vi "process board dll.vi"(8 "error in (no error)":errorcluster, 11 "board":i8) -> (0 "error out":errorcluster, 3 "board out":i8)   [LabVIEW 2025, in "uncoverspace.lvlib"]
doc: "void process_board_dll(int8_t board[Z][Y][X]);\nvoid process_board_dll(int8_t *board);"
uses:
  uncoverspace.lvlib
  uncoverspace.dll
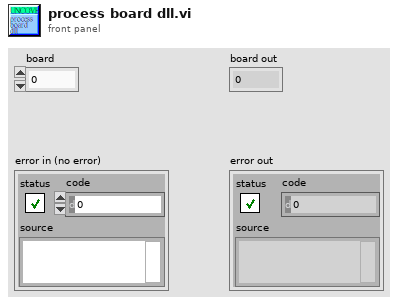
[diagram p1: front panel]
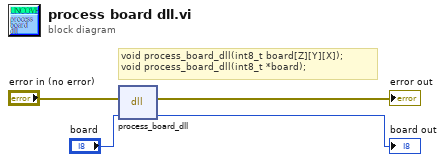
[diagram p0: block diagram]
diagram:
  # "void process_board_dll(int8_t board[Z][Y][X]);\nvoid process_board_dll(int8_t *board);"
  n1 = dll-call lib="C:/Users/daimapi/Desktop/project/minesweeper/c_code/uncoverspace/uncoverspace.*" fn="process_board_dll"(error in="error in (no error)", "board"="board") -> (error out=→"error out":errorcluster, "board"=→"board out":i8)  [unwired: 3 in, 1 out]
